vi "joinStyle.vi"(8 "Error In":errorcluster, 11 "QPen In":refnum<class "QPen.lvclass">) -> (0 "Error Out":errorcluster, 2 "Value":T1 items=["MiterJoin"=0, "BevelJoin"=64, "RoundJoin"=128, "SvgMiterJoin"=256, "MPenJoinStyle"=448], 3 "QPen Out":refnum<class "QPen.lvclass">)   [LabVIEW 2014, in "QPen.lvclass"]
doc: "LabVIEW-specific documentation is not yet available. See <b>https://doc.qt.io/qt-5/qpen.html#joinStyle</b>"
uses:
  QPen.lvclass
  LQ Core/Qt/PenJoinStyle.ctl
  LQ Core/LQSerialData/LQSerialData.lvclass/LQSerialData.ctl
  LQ Core/LQ Core.lvlib
  LQ Core/LQSerialData/LQSerialData.lvclass
  LQ Core/Qt/Qt.lvlib
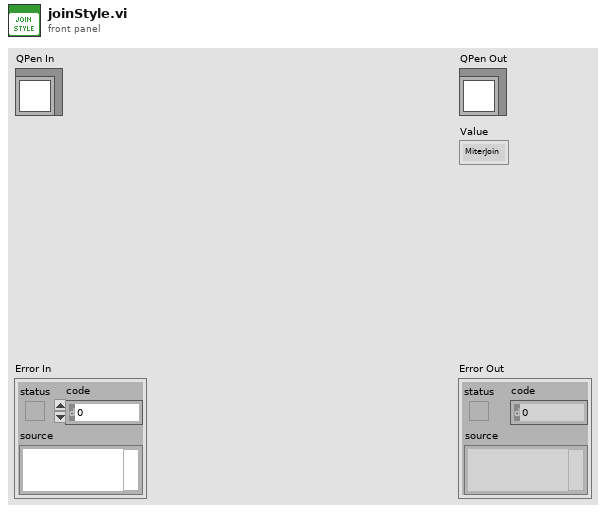
[diagram p1: front panel]
types:
  T1 = typedef "Qt.lvlib/PenJoinStyle.ctl" = i32
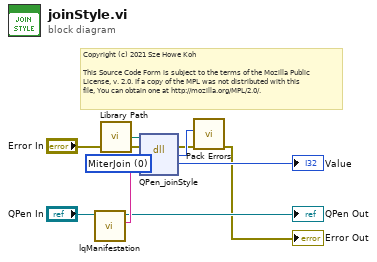
[diagram p0: block diagram]
diagram:
  w8 = T1 0 items=["MiterJoin"=0, "BevelJoin"=64, "RoundJoin"=128, "SvgMiterJoin"=256, "MPenJoinStyle"=448] ("retVal")
  # "Copyright (c) 2021 Sze Howe Koh\n\nThis Source Code Form is subject to the terms of the Mozilla Public\nLicense, v. 2.0. If a copy of the MPL was not distributed with this\nfile, You can obtain one at http://mozilla.org/MPL/2.0/."
  n1 = call "lqManifestation.vi"("LQSerialData in"="QPen In") -> ("Manifestation"=w7:string, "LQSerialData out"=→"QPen Out":refnum<class "QPen.lvclass">)  [unwired: 9 in]
  n2 = call "Library Path.vi"() -> ("Library Path"=w4:path)
  n3 = dll-call lib="?" fn="QPen_joinStyle"(path in=w4, error in="Error In", "_retVal"=w8, "_instance"=w7) -> (error out=w2:errorcluster, w3:i32, "_retVal"=→"Value":i32)  [unwired: 2 in, 1 out]
  n4 = call "Pack Errors.vi"("Error In"=w2, "Error Code"=w3) -> ("Error Out"=→"Error Out":errorcluster)  [unwired: 9 in]
